vi "000 Case exemple.vi"() -> ()   [LabVIEW 2019]
panel:
  out "Numeric 4":dbl
  in  "Numeric 3":dbl
  out "Numeric 2":dbl
  out "Numeric":dbl
  in  "Boolean":bool
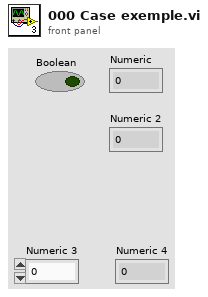
[diagram p1: front panel]
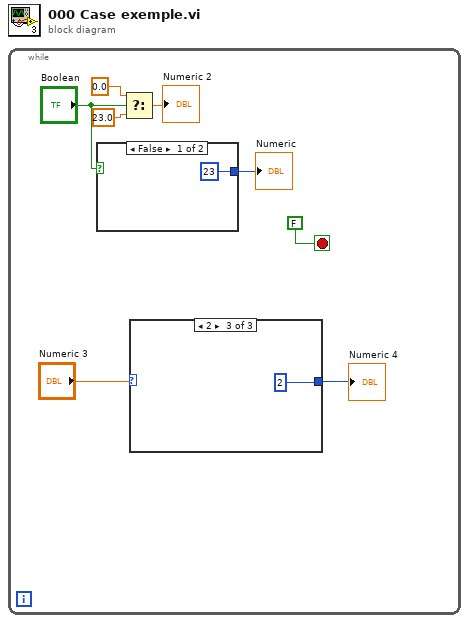
[diagram p0: block diagram]
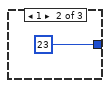
[diagram p3: hidden frame]
diagram:
  n1 = while {
    stop <- FALSE stop-if-true
    n2 = case shown="False" "Boolean" {
      tunnel: [23 _] -> w8
      frame False {
      }
      frame True {
      }
    }
    "Numeric" <- w8
    n3 = Select(t=0.0, s="Boolean", f=23.0) -> (s? t:f=→"Numeric 2":dbl)
    n4 = case shown="2" "Numeric 3" {
      tunnel: [_ 23 2] -> w1
      frame 0, Default {
      }
      frame 1 {
      }
      frame 2 {
      }
    }
    "Numeric 4" <- w1
  }
